vi "G4BaseTemplate_Simple_5x6x5_ReadProperty.vi"(0 "reference in":refnum<class "G4BaseTemplate_Simple_5x6x5.lvclass">, 11 "error in (no error)":errorcluster) -> (4 "reference out":refnum<class "G4BaseTemplate_Simple_5x6x5.lvclass">, 8 "property":dbl, 15 "error out":errorcluster)   [LabVIEW 2014]
uses:
  <resource>/Framework/Providers/Open_GDS/ClassProviders/Provider_EndevoGOOP400/Templates/G4BaseTemplate_Simple_5x6x5/G4BaseTemplate_Simple_5x6x5.lvclass
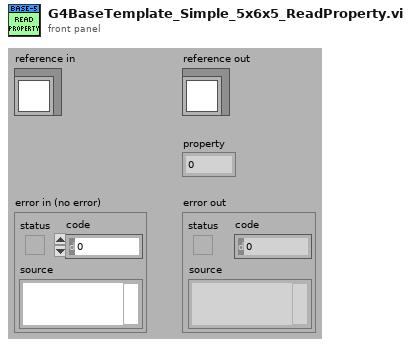
[diagram p1: front panel]
types:
  T1 = typedef "G4BaseTemplate_Simple_5x6x5.lvclass/ObjectAttributes.ctl" = cluster{"Attribute1":dbl}
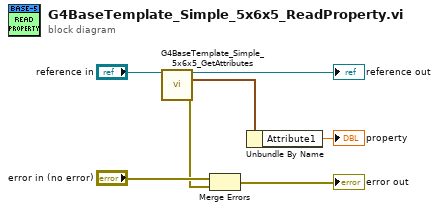
[diagram p0: block diagram]
diagram:
  n1 = call <resource>:"G4BaseTemplate_Simple_5x6x5_GetAttributes.vi"("reference in"="reference in") -> ("reference out"=→"reference out":refnum<class "G4BaseTemplate_Simple_5x6x5.lvclass">, "Data"=w4:T1, "error out"=w2:errorcluster)  [unwired: 11 in, 1 out]
  n2 = Merge Errors("error in (no error)", w2) -> (→"error out":errorcluster)
  n3 = Unbundle By Name(w4) -> ("Attribute1"=→"property":dbl)
